vi "GetControlRef.vi"(8 "error in (no error)":errorcluster, 10 "Control Label":string, 11 "VI Reference":refnum<vi>) -> (0 "error out":errorcluster, 3 "Ctl Refnum":refnum<vi>)   [LabVIEW 2019]
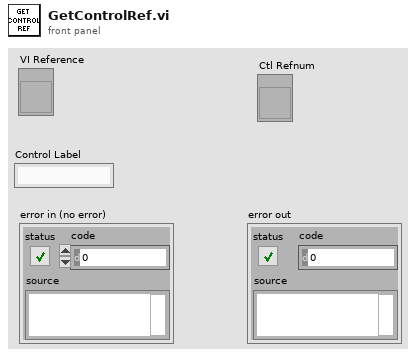
[diagram p1: front panel]
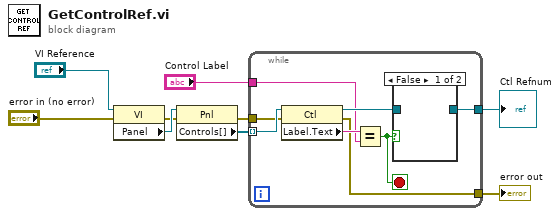
[diagram p0: block diagram]
diagram:
  n1 = property class="VI"(reference="VI Reference", error in="error in (no error)") -> (error out=w8:errorcluster, "Panel"=w9:refnum<vi>)  [unwired: 1 out]
  n2 = property class="Pnl"(reference=w9, error in=w8) -> (error out=w3:errorcluster, "Controls[]"=w7:refnum<vi>[])  [unwired: 1 out]
  n3 = while {
    tunnel: w7 -> [w17] mode=indexing
    tunnel: "Control Label" -> [w14]
    tunnel: w3 -> [w12]
    tunnel: [w11] -> w2
    tunnel: [w10] -> w1
    stop <- w13 stop-if-true
    n4 = property class="Ctl"(reference=w17, error in=w12) -> (reference out=w16:refnum<vi>, error out=w11:errorcluster, "Label.Text"=w15:string)
    n5 = Equal?(x=w15, y=w14) -> (x = y?=w13:bool)
    n6 = case shown="False" w13 {
      tunnel: w16 -> [_ w18]
      tunnel: [_ w18] -> w10
      frame False {
      }
      frame True {
      }
    }
  }
  "error out" <- w2
  "Ctl Refnum" <- w1
